vi "Read Variant.vi"(8 "error in (no error)":errorcluster, 10 "Tag":string, 11 "Var Bus in":refnum<class "Omni_Bus.lvclass">) -> (0 "error out":errorcluster, 2 "Variant":variant, 3 "Var Bus out":refnum<class "Omni_Bus.lvclass">)   [LabVIEW 2021, in "Omni_Bus.lvclass"]
uses:
  Omni_Bus.lvclass
  <vilib>/TSA/Abstract Data Classes/Abs_Types/Variant/Abs_Variant.lvclass
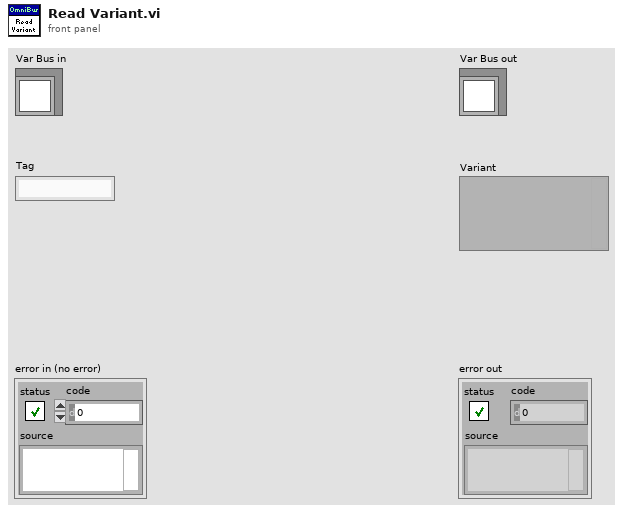
[diagram p1: front panel]
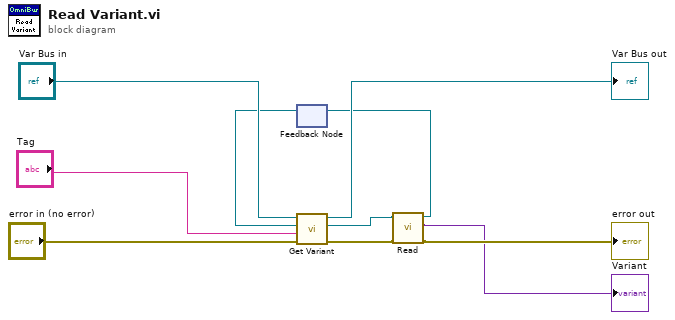
[diagram p0: block diagram]
diagram:
  n1 = feedback #1() -> (w6:refnum<class "Abs_Variant.lvclass">)  [unwired: 1 in]
  n2 = call-dynamic "Get Variant.vi"("error in (no error)"="error in (no error)", "Tag"="Tag", "Value Type"=w6, "Var Bus in"="Var Bus in") -> ("error out"=w5:errorcluster, "Value Out"=w4:refnum<class "Abs_Variant.lvclass">, "Var Bus out"=→"Var Bus out":refnum<class "Omni_Bus.lvclass">)  [unwired: 5 in]
  n3 = call-dynamic "Read.vi"("error in (no error)"=w5, "Abs_Variant in"=w4) -> ("error out"=→"error out":errorcluster, "Variant"=→"Variant":variant, "Abs_Variant out"=w2:refnum<class "Abs_Variant.lvclass">)  [unwired: 7 in]
  n4 = feedback-in #1(w2) -> ()
